vi "Is output settled.vi"(8 "error in (no error)":errorcluster, 11 "Settle Output in":refnum<class "Settle Output.lvclass">) -> (0 "error out":errorcluster, 2 "Is output settled?":bool, 3 "Settle Output out":refnum<class "Settle Output.lvclass">)   [LabVIEW 2015, in "Settle Output.lvclass"]
uses:
  Settle Output.lvclass
  Settle Output.lvclass/Settle Output.ctl
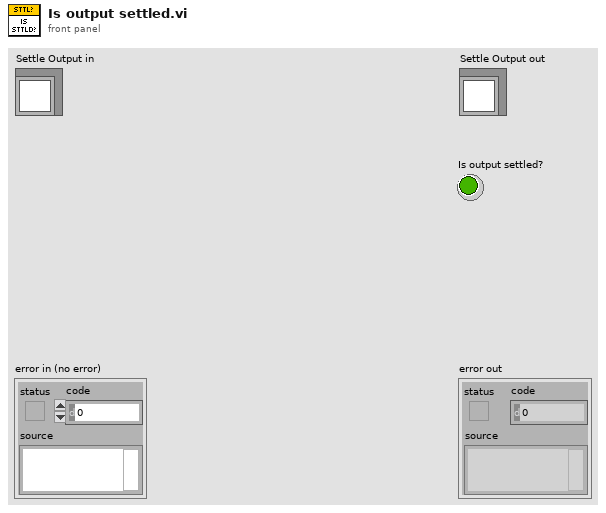
[diagram p1: front panel]
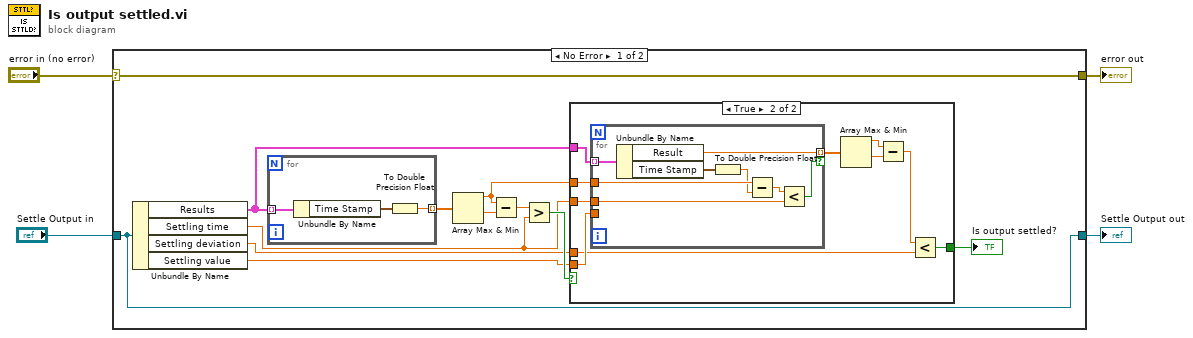
[diagram p0: block diagram]
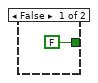
[diagram p2: hidden frame]
diagram:
  n1 = case shown="No Error" "error in (no error)" {
    selector: "error in (no error)" -> [w5 w40]
    tunnel: [w5 w40] -> w3
    tunnel: [w16 w39] -> w1
    tunnel: "Settle Output in" -> [w16 w39]
    frame No Error {
      n2 = Unbundle By Name(w16) -> ("Results"=w11:cluster{"Time Stamp":timestamp, "Result":dbl}[], "Settling time"=w10:dbl, "Settling deviation"=w6:dbl, "Settling value"=w8:dbl)
      n3 = for {
        tunnel: w11 -> [w38] mode=indexing
        tunnel: [w36] -> w12 mode=indexing
        n4 = Unbundle By Name(w38) -> ("Time Stamp"=w37:timestamp)
        n5 = To Double Precision Float(number=w37) -> (double precision float=w36:dbl)
      }
      n6 = Array Max & Min(array=w12) -> (max value=w9:dbl, min value=w15:dbl)  [unwired: 2 out]
      n7 = Subtract(x=w9, y=w15) -> (x-y=w14:dbl)
      n8 = Greater?(x=w14, y=w10) -> (0:w13:bool)
      n9 = case shown="True" w13 {
        tunnel: w11 -> [_ w27]
        tunnel: w10 -> [_ w26]
        tunnel: w9 -> [_ w25]
        tunnel: w8 -> [_ w24]
        tunnel: [FALSE w18] -> w7
        tunnel: w6 -> [_ w19]
        frame False {
        }
        frame True {
          n10 = for {
            tunnel: w27 -> [w34] mode=indexing
            tunnel: w26 -> [w35]
            tunnel: w25 -> [w32]
            tunnel: w24 -> [_]
            tunnel: [w28] -> w23 mode=indexing if=w29
            n11 = Unbundle By Name(w34) -> ("Result"=w28:dbl, "Time Stamp"=w33:timestamp)
            n12 = To Double Precision Float(number=w33) -> (double precision float=w31:dbl)
            n13 = Subtract(x=w32, y=w31) -> (x-y=w30:dbl)
            n14 = Less?(x=w30, y=w35) -> (x < y?=w29:bool)
          }
          n15 = Array Max & Min(array=w23) -> (max value=w21:dbl, min value=w22:dbl)  [unwired: 2 out]
          n16 = Subtract(x=w21, y=w22) -> (x-y=w20:dbl)
          n17 = Less?(x=w20, y=w19) -> (x < y?=w18:bool)
        }
      }
      "Is output settled?" <- w7
    }
    frame Error {
    }
  }
  "error out" <- w3
  "Settle Output out" <- w1
